vi "MaxPIDDriv.vi"(6 "Reset":bool, 8 "dt (s)":dbl, 11 "Error":dbl) -> (3 "Drivative":dbl)   [LabVIEW 2012]
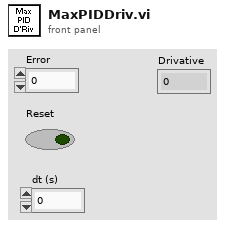
[diagram p1: front panel]
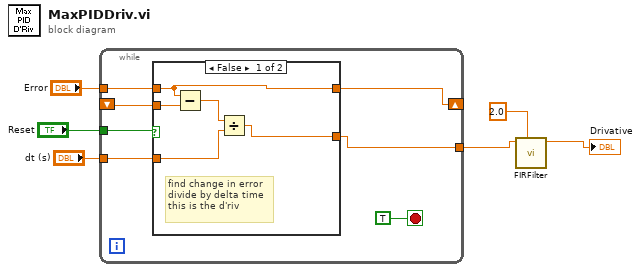
[diagram p0: block diagram]
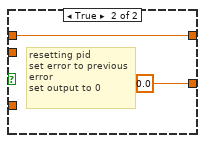
[diagram p2: hidden frame]
diagram:
  n1 = while {
    tunnel: "Error" -> [w12]
    tunnel: "Reset" -> [w11]
    tunnel: "dt (s)" -> [w10]
    shift-right: [w9] -> _
    shift-left: _ -> [w8]
    tunnel: [w7] -> w3
    stop <- TRUE stop-if-true
    n2 = case shown="False" w11 {
      tunnel: w12 -> [w16 w19]
      tunnel: w10 -> [w18 _]
      tunnel: [w14 0.0] -> w7
      tunnel: [w16 w19] -> w9
      tunnel: w8 -> [w15 _]
      frame False {
        # "find change in error\ndivide by delta time\nthis is the d'riv"
        n3 = Subtract(x=w16, y=w15) -> (x-y=w17:dbl)
        n4 = Divide(x=w17, y=w18) -> (x/y=w14:dbl)
      }
      frame True {
        # "resetting pid\nset error to previous\nerror\nset output to 0"
      }
    }
  }
  n5 = call "FIRFilter.vi"("Filter Size"=2.0, "Input"=w3) -> ("Output"=→"Drivative":dbl)  [unwired: 9 in]
